vi "setChannel.vi"(8 "error in (no error)":errorcluster, 9 "Channel":refnum<class "Channel.lvclass">, 10 "index":i32, 11 "ChannelArray.lvclass in":refnum<class "ChannelArray.lvclass">) -> (0 "error out":errorcluster, 3 "ChannelArray.lvclass out":refnum<class "ChannelArray.lvclass">)   [LabVIEW 2009, in "Tools.lvlib" / "DatabaseHelpers.lvlib" / "ChannelArray.lvclass"]
uses:
  ChannelArray.lvclass
  Channel/Channel.lvclass
  ChannelArray.lvclass/ChannelArray.ctl
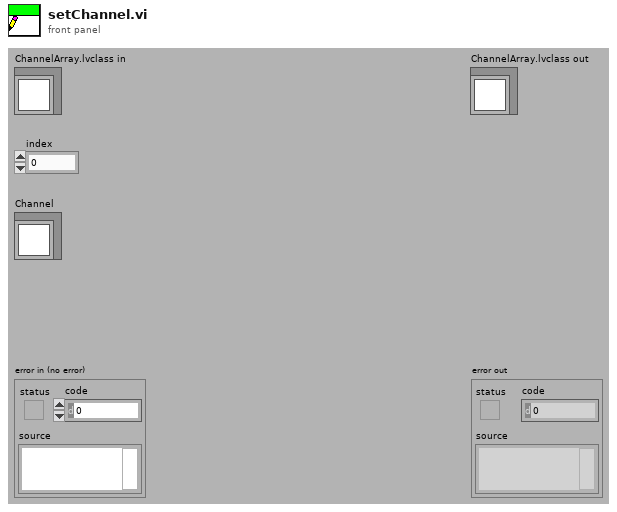
[diagram p1: front panel]
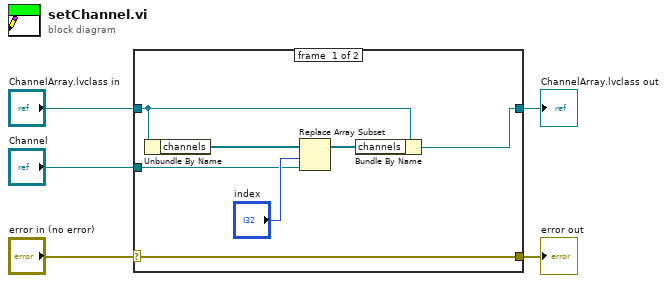
[diagram p0: block diagram]
diagram:
  n1 = case shown="No Error" "error in (no error)" {
    selector: "error in (no error)" -> [w12 w13]
    tunnel: [w12 w13] -> w4
    tunnel: [w11 w14] -> w2
    tunnel: "ChannelArray.lvclass in" -> [w10 w14]
    tunnel: "Channel" -> [w6 _]
    frame #0 {
      n2 = Unbundle By Name(w10) -> ("channels"=w9:refnum<class "Channel.lvclass">[])
      n3 = Replace Array Subset(array=w9, new element=w6, index="index") -> (w8:refnum<class "Channel.lvclass">[])
      n4 = Bundle By Name(cluster=w10, "channels"=w8) -> (w11:refnum<class "ChannelArray.lvclass">)
    }
    frame #1 {
    }
  }
  "error out" <- w4
  "ChannelArray.lvclass out" <- w2
